vi "Event from Ring.vi"(7 "Time Stamp":timestamp, 10 "Value":refnum<vi>, 11 "VI Refnum":refnum<vi>) -> (2 "Event Data":T1)   [LabVIEW 2023, in "Instruments.lvlib" / "Instruments.lvclass"]
uses:
  Library/Instruments.lvclass
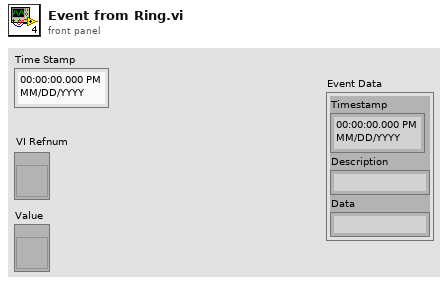
[diagram p1: front panel]
types:
  T1 = cluster{"Timestamp":timestamp, "Description":string, "Data":string}
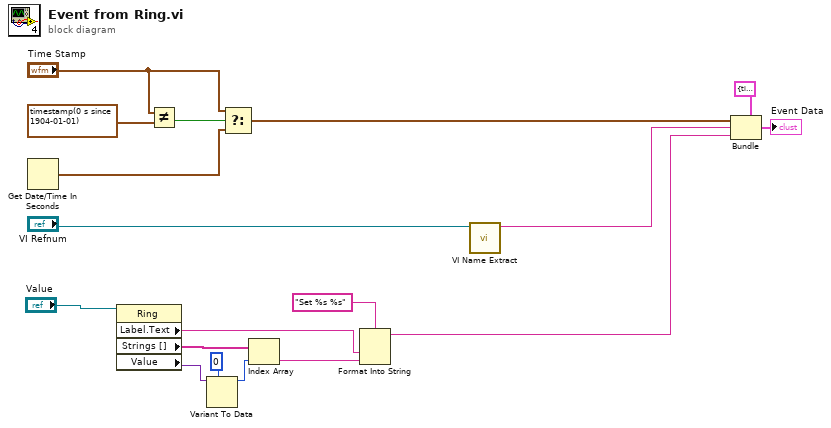
[diagram p0: block diagram]
diagram:
  n1 = Get Date/Time In Seconds() -> (seconds since 1Jan1904=w13:timestamp)
  n2 = property class="Ring"(reference="Value") -> ("Label.Text"=w4:string, "Strings []"=w10:string[], "Value"=w9:variant)  [unwired: 1 in, 2 out]
  n3 = Not Equal?(x="Time Stamp", y=timestamp(0 s since 1904-01-01) ("Time Stamp")) -> (x != y?=w15:bool)
  n4 = Variant To Data(type=0, Variant=w9) -> (data=w7:i32)  [unwired: 1 in, 1 out]
  n5 = Select(t="Time Stamp", s=w15, f=w13) -> (s? t:f=w12:timestamp)
  n6 = Index Array(array=w10, index=w7) -> (element=w5:string)
  n7 = Format Into String(format string="Set %s %s", w4, w5) -> (resulting string=w6:string)  [unwired: 2 in, 1 out]
  n8 = call "VI Name Extract.vi"("VI Refnum"="VI Refnum") -> ("Name"=w1:string)  [unwired: 10 in]
  n9 = Bundle(cluster=T1 {"Timestamp"=timestamp(0 s since 1904-01-01), "Description"="", "Data"=""}, "Timestamp"=w12, "Description"=w1, "Data"=w6) -> (→"Event Data":T1)
